vi "DashboardSetOperationalMode.vi"(8 "Dashboard":refnum<k24>, 9 "mode":i32(ring) items=["Manual", "Automatic", "None"], 11 "error in":errorcluster) -> (0 "Response":cluster{"Message":string, "Succeed":bool}, 3 "error out":errorcluster)   [LabVIEW 2022 SP3, in "UnderAutomation.UniversalRobots.lvlib"]
uses:
  UnderAutomation.UniversalRobots.lvlib
  C:/Users/fg/Documents/UniversalRobots.vi/LabVIEW_2023/UnderAutomation.UniversalRobots/lib/UnderAutomation.UniversalRobots.dll
  LabVIEW_2023/UnderAutomation.UniversalRobots/lib/UnderAutomation.UniversalRobots.dll
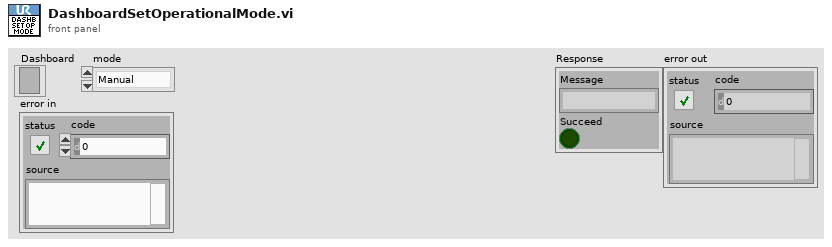
[diagram p1: front panel]
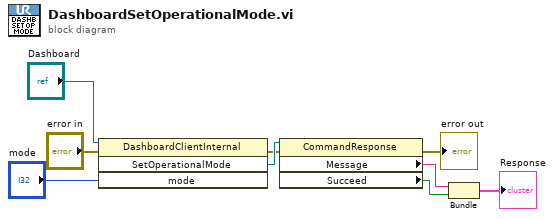
[diagram p0: block diagram]
diagram:
  n1 = invoke class="DashboardClientInternal" method="SetOperationalMode"(reference="Dashboard", error in="error in", "mode"="mode") -> (error out=w3:errorcluster, "SetOperationalMode"=w8:refnum<k24>)  [unwired: 1 in, 2 out]
  n2 = property class="CommandResponse"(reference=w8, error in=w3) -> (error out=→"error out":errorcluster, "Message"=w7:string, "Succeed"=w6:bool)  [unwired: 1 out]
  n3 = Bundle("Message"=w7, "Succeed"=w6) -> (→"Response":cluster{"Message":string, "Succeed":bool})  [unwired: 1 in]
